vi "视觉手动.vi"() -> ()   [LabVIEW 2015]
uses:
  <vilib>/vision/driver/NI_Vision_Acquisition_Software.lvlib
  <vilib>/vision/driver/IMAQdx.llb/IMAQdx Acquisition Mode.ctl
  <vilib>/userdefined/High Color/IMAQdx.ctl
  <vilib>/vision/driver/IMAQdx.llb/IMAQdx Buffer Number Mode.ctl
  Global.vi
panel:
  out "String (OCR/OCV 1)":string
  in  "建立模板":bool
  out "Image":T1(plugin-control)
  in  "拍照":bool
  in  "打开光源":bool
  in  "停止":bool
  # "遥控器增加模板手动操作"
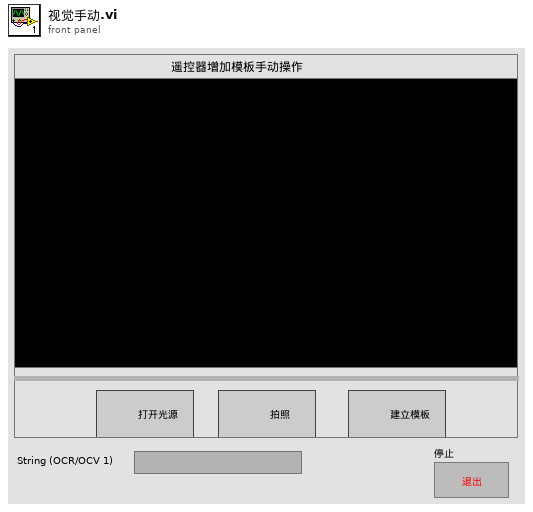
[diagram p1: front panel]
types:
  T1 = typedef "IMAQ Image.ctl" = refnum<image>
  T2 = typedef "IMAQdx.ctl" = refnum<k21>
  T3 = typedef "NI_Vision_Acquisition_Software.lvlib/IMAQdx Acquisition Mode.ctl" = enum32{"One Shot", "Continuous"}
  T4 = typedef "NI_Vision_Acquisition_Software.lvlib/IMAQdx Buffer Number Mode.ctl" = enum32{"Next", "Last", "Buffer Number", "Every", "Last New"}
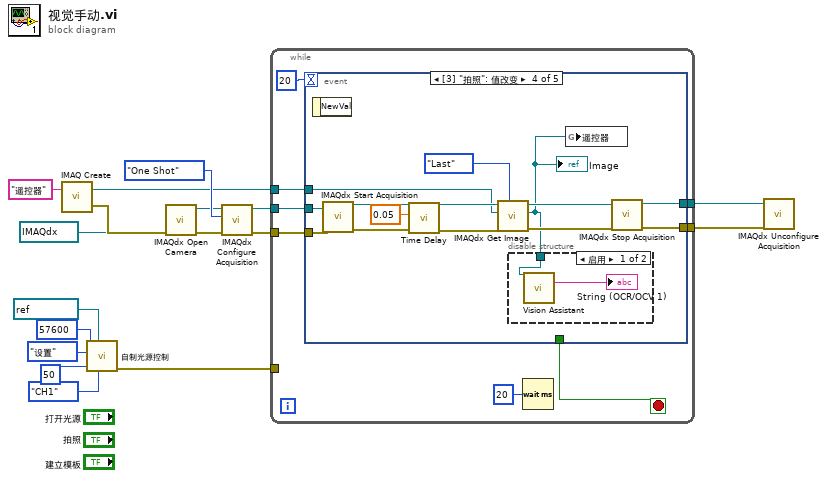
[diagram p0: block diagram]
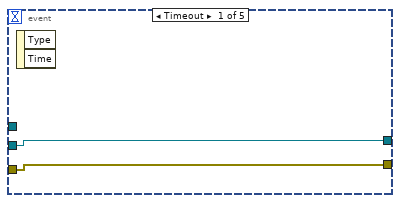
[diagram p2: hidden frame]
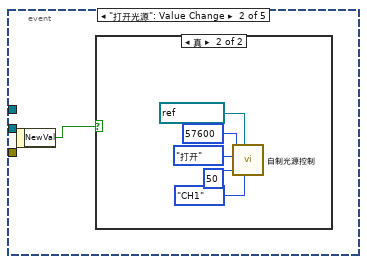
[diagram p3: hidden frame]
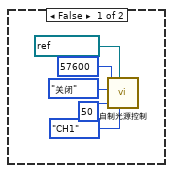
[diagram p4: hidden frame]
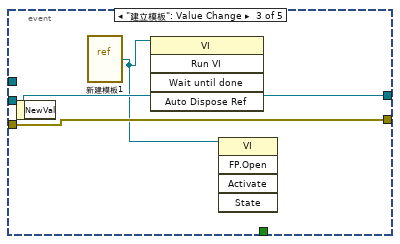
[diagram p5: hidden frame]
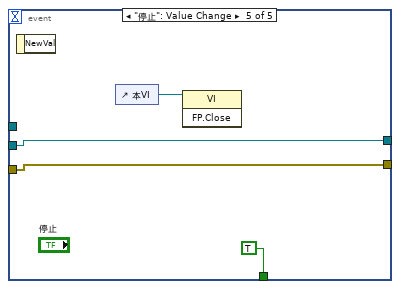
[diagram p7: hidden frame]
diagram:
  n1 = call "IMAQ Create"("Image Name"="遥控器") -> ("New Image"=w3:T1, "error out"=w13:errorcluster)  [unwired: 3 in, 1 out]
  n2 = call "自制光源控制.vi"("通道"=enum16{"CH1", "CH2", "CH3", "CH4"}."CH1", "VISA In"=refnum<visa-resource-name> "COM2", "亮度"=50 ("亮度值"), "操作模式"=enum16{"打开", "关闭", "设置"}."设置", "baud rate"=u32 57600) -> ("错误输出"=w6:errorcluster)  [unwired: 4 in, 2 out]
  n3 = call <vilib>:"IMAQdx Open Camera.vi"("error in"=w13, "Session In"=T2 "cam0") -> ("error out"=w17:errorcluster, "Session Out"=w15:T2)  [unwired: 1 in, 7 out]
  n4 = call <vilib>:"IMAQdx Configure Acquisition.vi"("error in"=w17, "Continuous?"=IMAQdx_Acquisition_Mode."One Shot", "Session In"=w15) -> ("error out"=w4:errorcluster, "Session Out"=w5:T2)  [unwired: 1 in, 6 out]
  n5 = while {
    tunnel: w6 -> [_]
    tunnel: w5 -> [w24]
    tunnel: w4 -> [w23]
    tunnel: w3 -> [w22]
    tunnel: [w21] -> w2
    tunnel: [w20] -> w1
    stop <- w18 stop-if-true
    n6 = event shown="[3] \"拍照\": 值改变" {
      selector: _ -> [_ _ _ _ _]
      dyn-events: _ -> [_ _ _ _ _]
      timeout: 20 -> [_ _ _ _ _]
      tunnel: w24 -> [w27 _ w41 w48 w59]
      tunnel: w23 -> [w26 _ w40 w47 w58]
      tunnel: w22 -> [_ _ _ w46 _]
      tunnel: [w27 _ w41 w45 w59] -> w21
      tunnel: [w26 _ w40 w44 w58] -> w20
      tunnel: [_ _ _ _ TRUE] -> w18
      event Timeout {
        n7 = event-data() -> ()  [unwired: 1 in, 2 out]
      }
      event "打开光源": Value Change {
        n8 = event-data() -> ("NewVal"=w28:bool)  [unwired: 1 in]
        n9 = case shown="真" w28 {
          frame False {
            n10 = call "自制光源控制.vi"("通道"=enum16{"CH1", "CH2", "CH3", "CH4"}."CH1", "VISA In"=refnum<visa-resource-name> "COM2", "亮度"=50 ("亮度值"), "操作模式"=enum16{"打开", "关闭", "设置"}."关闭", "baud rate"=u32 57600) -> ()  [unwired: 4 in, 3 out]
          }
          frame True {
            n11 = call "自制光源控制.vi"("通道"=enum16{"CH1", "CH2", "CH3", "CH4"}."CH1", "VISA In"=refnum<visa-resource-name> "COM2", "亮度"=50 ("亮度值"), "操作模式"=enum16{"打开", "关闭", "设置"}."打开", "baud rate"=u32 57600) -> ()  [unwired: 4 in, 3 out]
          }
        }
      }
      event "建立模板": Value Change {
        n12 = event-data() -> ()  [unwired: 1 in, 1 out]
        n13 = vi-ref "新建模板1.vi"() -> (w39:refnum<vi>)
        n14 = invoke class="VI" method="Run VI"(reference=w39) -> ()  [unwired: 4 in, 5 out]
        n15 = invoke class="VI" method="FP.Open"(reference=w39) -> ()  [unwired: 4 in, 5 out]
      }
      event "拍照": Value Change {
        n16 = event-data() -> ()  [unwired: 1 in, 1 out]
        n17 = call <vilib>:"IMAQdx Start Acquisition.vi"("error in"=w47, "Session In"=w48) -> ("error out"=w51:errorcluster, "Session Out"=w54:T2)  [unwired: 8 out]
        n18 = call "Time Delay"("error in (no error)"=w51, "Delay Time (s)"=0.05) -> ("error out"=w53:errorcluster)  [unwired: 9 in]
        n19 = call <vilib>:"IMAQdx Get Image.vi"("Buffer Number Mode (Next)"=IMAQdx_Buffer_Number_Mode."Last", "error in"=w53, "Image In"=w46, "Session In"=w54) -> ("error out"=w50:errorcluster, "Image Out"=w42:T1, "Session Out"=w49:T2)  [unwired: 1 in, 4 out]
        "Image" <- w42
        n20 = disable-structure shown="启用" {
          disable-tunnel: w42 -> [w55 _]
          frame Enabled {
            n21 = call "Vision Assistant"("Image In"=w55) -> ("String (OCR/OCV 1)"=→"String (OCR/OCV 1)":string)  [unwired: 23 in, 3 out]
          }
          frame Disabled {
          }
        }
        n22 = global write "Global.vi" "遥控器"(w42) -> ()
        n23 = call <vilib>:"IMAQdx Stop Acquisition.vi"("error in"=w50, "Session In"=w49) -> ("error out"=w44:errorcluster, "Session Out"=w45:T2)  [unwired: 8 out]
      }
      event "停止": Value Change {
        n24 = event-data() -> ()  [unwired: 1 in, 1 out]
        n25 = control-ref of="本VI"() -> (w57:refnum<vi>)
        n26 = invoke class="VI" method="FP.Close"(reference=w57) -> ()  [unwired: 2 in, 3 out]
      }
    }
    n27 = Wait (ms)(milliseconds to wait=u32 20 ("等待时间（毫秒）")) -> ()  [unwired: 1 out]
  }
  n28 = call <vilib>:"IMAQdx Unconfigure Acquisition.vi"("error in"=w1, "Session In"=w2) -> ()  [unwired: 10 out]
